vi "PathMathTest.vi"() -> ()   [LabVIEW 2018]
panel:
  out "current pt 2":i32
  in  "current pt":i32
  out "Result":dbl[][](array[numeric])
  out "All Data (index by column)":dbl[][](array[numeric])
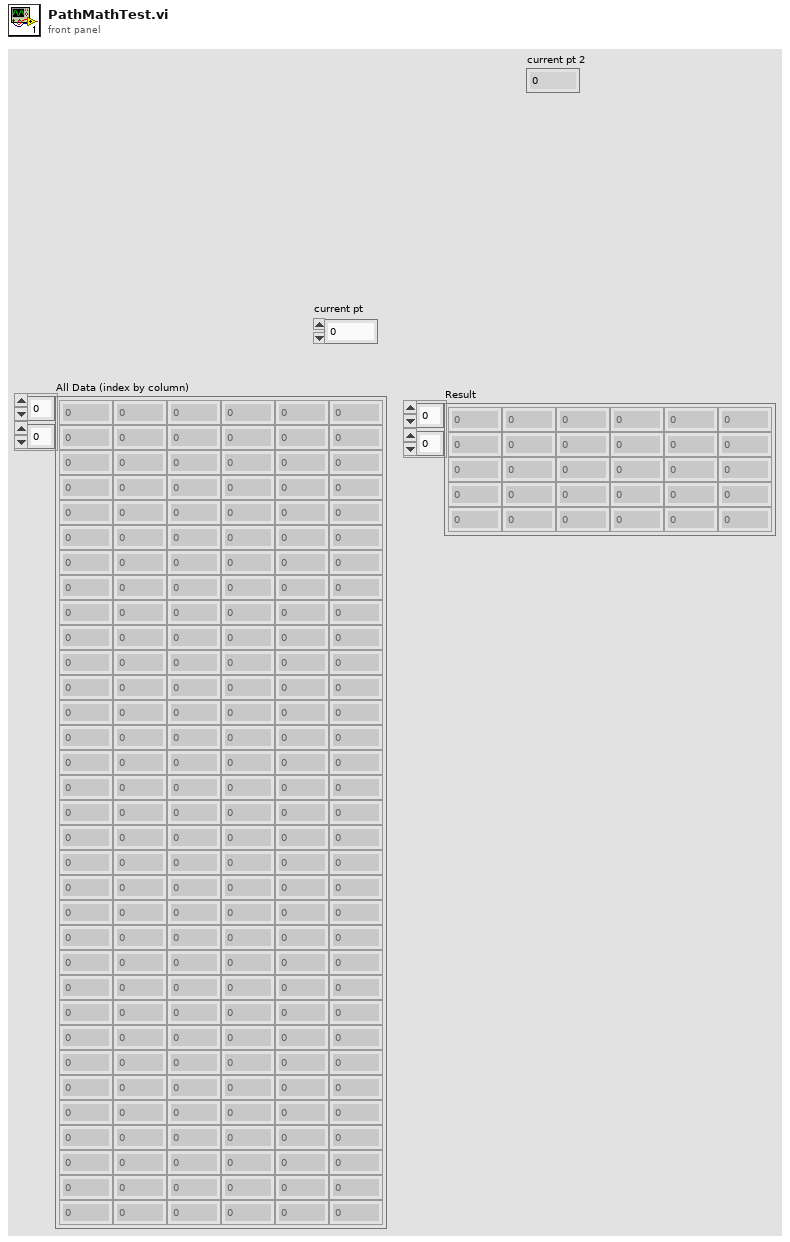
[diagram p1: front panel]
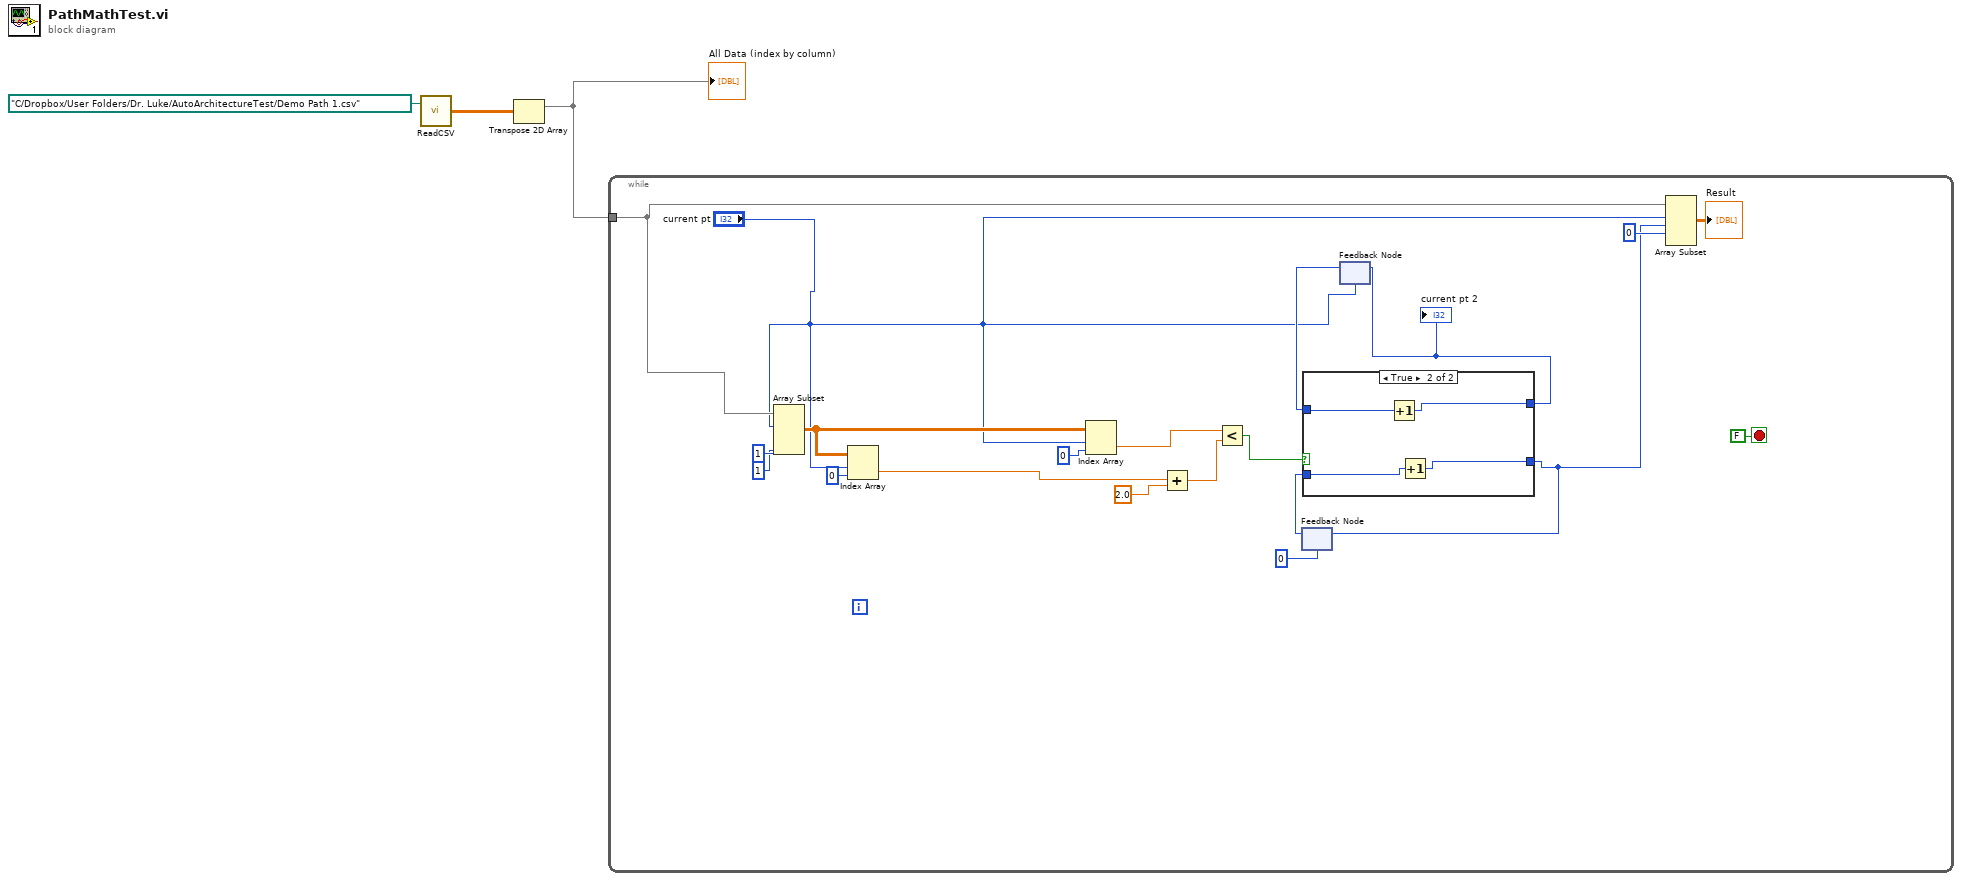
[diagram p0: block diagram]
diagram:
  n1 = call "ReadCSV.vi"("File Path (.csv)"=path "C:/Dropbox/User Folders/Dr. Luke/AutoArchitectureTest/Demo Path 1.csv") -> ("Data (index by column)"=w2:dbl[][])  [unwired: 1 in]
  n2 = Transpose 2D Array(2D array=w2) -> (transposed array=w1:dbl[][])
  "All Data (index by column)" <- w1
  n3 = while {
    tunnel: w1 -> [w18]
    stop <- FALSE stop-if-true
    n4 = Array Subset(array=w18, index (row)="current pt", index (col)=1 ("index"), length (col)=1 ("length")) -> (w17:dbl[][])  [unwired: 1 in]
    n5 = Index Array(array=w17, index (row)="current pt", index (col)=0 ("disabled index (col)")) -> (element=w16:dbl)
    n6 = Index Array(array=w17, index (row)="current pt", index (col)=0 ("disabled index (col)")) -> (element=w9:dbl)
    n7 = Add(x=w16, y=2.0) -> (x+y=w11:dbl)
    n8 = Less?(x=w9, y=w11) -> (x < y?=w10:bool)
    n9 = feedback #1(0) -> (w7:i32)
    n10 = feedback #2("current pt") -> (w5:i32)
    n11 = case shown="True" w10 {
      tunnel: w5 -> [w25 w29]
      tunnel: [w25 w28] -> w6
      tunnel: [w24 w27] -> w14
      tunnel: w7 -> [w24 w26]
      frame False {
      }
      frame True {
        n12 = Increment(x=w29) -> (x+1=w28:i32)
        n13 = Increment(x=w26) -> (x+1=w27:i32)
      }
    }
    "current pt 2" <- w6
    n14 = feedback-in #1(w14) -> ()
    n15 = feedback-in #2(w6) -> ()
    n16 = Array Subset(array=w18, index (row)="current pt", length (row)=w14, index (col)=0 ("index")) -> (→"Result":dbl[][])  [unwired: 1 in]
  }
